vi "Write ExperimentVariables.vi"(10 "ExperimentVariables.lvclass":refnum<class "ExperimentVariables.lvclass">, 11 "Experiment in":refnum<class "Experiment.lvclass">) -> (3 "Experiment out":refnum<class "Experiment.lvclass">)   [LabVIEW 2013]
uses:
  Experiment.lvclass
  ExperimentVariables/ExperimentVariables.lvclass
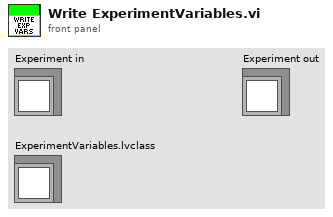
[diagram p1: front panel]
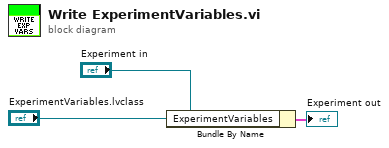
[diagram p0: block diagram]
diagram:
  n1 = Bundle By Name(cluster="Experiment in", "ExperimentVariables"="ExperimentVariables.lvclass") -> (→"Experiment out":cluster{})
